vi "BusController.vi"() -> ()   [LabVIEW 2017, in "BusController.lvlib"]
uses:
  BusController.lvlib
  Admin/BCAdmin.lvclass
  Admin/BCAdmin.lvclass/BCAdmin.ctl
  Queue/QueueType.ctl
  Bus_class/Private/BdcstInfo.ctl
  Bus_class/Private/ModuleType.ctl
  Bus_class/Public/TypeDefs/clBusData.ctl
  FrontPanel/TypeDefs/clEventConfig.ctl
  Modules/PmuImpairPlugins/PmuImpairPluginBase_class/TypeDefs/clImpairConfig.ctl
  Modules/EventPlugins/EventPluginBaseClass/TypeDefs/clEvtReportArray.ctl
  Modules/EventPlugins/EventPluginBaseClass/TypeDefs/clEvtReport.ctl
  Modules/EventPlugins/EventPluginBaseClass/TypeDefs/dblEvtSignalArray.ctl
  Modules/NetworkImpairmentModule/PublicAPI/Arguments/Broadcasts/dblNetworkTime.ctl
  Modules/NetworkImpairmentModule/PublicAPI/Arguments/Broadcasts/dblPktLoss.ctl
  Modules/FlagImpairModule/PublicAPI/Arguments/Broadcasts/ui32FlagImpairmentArray.ctl
  Modules/OutputToFilePlugins/OutputToFileBasePlugin/Typedefs/PmuCfgOpt.ctl
  Admin/Accessors/Read ShowPanel_.vi
  Admin/Accessors/Read BC ID.vi
  Admin/Accessors/Read Name.vi
  Admin/Read Script.vi
  Admin/Accessors/Read BusIndex.vi
  Admin/Accessors/Read First_.vi
  Admin/Read BcQueName.vi
  Admin/Accessors/Read BCRegRef.vi
  <vilib>/Utility/error.llb/Error Cluster From Error Code.vi
  <vilib>/Analysis/1siggen.llb/Ramp Pattern by Delta.vi
  <vilib>/ErrorRing/Error Ring.xnode
  Admin/Registry/BCReg.lvclass
  Bus_class/Bus.lvclass
  <userlib>/NIST/NISTErrorLib/NISTErrorLib.lvlib
  Framework.lvlib
  Modules/PmuImpairPlugins/PmuImpairPluginBase_class/PmuImpairPluginBase.lvclass
  Modules/EventPlugins/EventPluginBaseClass/EventPluginBaseClass.lvclass
  Modules/NetworkImpairmentModule/NetworkImpairmentModule.lvlib
  Modules/FlagImpairModule/FlagImpairModule.lvlib
  Modules/OutputToFilePlugins/OutputToFileBasePlugin/OutputToFileBasePlugin.lvclass
  Modules/EventModule/EventModule.lvlib
  <vilib>/Analysis/NI_AALBase.lvlib
  Modules/PmuImpairModule/PmuImpairModule.lvlib
  ModuleType.ctl
panel:
  out "LastCommand":string
  out "Script":string[](array[string])
  out "BcQueName":string
  out "BC ID":i32
  out "First_":bool
  in  "BCAdmin":refnum<class "BCAdmin.lvclass">
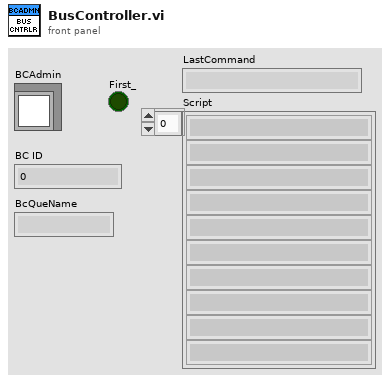
[diagram p1: front panel]
types:
  T1 = typedef "Framework.lvlib/clFrameworkData.ctl" = cluster{"EvtINIFilePaths":path[], "BusClassInstances":refnum<class "Bus.lvclass">[], "PmuImpairINIFilePaths":path[], "FlagImpairINIFilePaths":path[], "NetImpairINIFilePaths":path[], "OutputToFileINIFilePaths":path[], "AppINIFilePaths":path[], "AppModuleID":i32, "OutputToFileID":i32}
  T2 = typedef "Bus_class.lvlib/Bus.lvclass/ModuleType.ctl" = enum16{"PMU", "Event", "Network", "Flag", "App", "OutToFile"}
  T3 = typedef "Bus_class.lvlib/Bus.lvclass/BdcstInfo.ctl" = cluster{"ModuleType":T2, "ModuleID":i32, "UsrEvtRef":variant, "ScriptCmd":string}
  T4 = typedef "BusController.lvlib/ModuleType.ctl" = enum16{"PMU", "Event", "Network", "Flag", "App"}
  T5 = enum32{"Invalid", "Standard", "Closed", "Hidden", "Minimized", "Maximized"}
  T6 = typedef "Bus_class.lvlib/Bus.lvclass/clBusData.ctl" = cluster{"BusNumber":u8, "EvtPluginINIFilePath":path, "EvtParams":string[][], "EvtConfig":T7, "Start Time":dbl, "End Time":dbl, "PmuImpairPluginINIFilePath":path, "PmuImpairParams ":string[][], "PmuImpairConfig":T8, "NetImpPluginINIFilePath":path, "NetImpParams":string[][], "FlagImpPluginINIFilePath":path, "FlagImpParams":string[][], "EvtReportArray":T9, "EventSignalArray":T11, "ImpairReportArray":T9, "NetworkTime":T12, "PktLoss":T13, "FlagImpArray":T14, "OutputToFilePluginINIFilePath":path, "Output File Path":path, "clConfigOptions":T15, "AppPluginINIFilePath":path, "AppConfig":variant, "AppOutput":variant}
  T7 = typedef "Framework.lvlib/clEventConfig.ctl" = cluster{"UTC Time 0":timestamp, "Nominal Frequency":u16, "Reporting Rate":u16, "Fsamp":u32, "PosSeq":bool}
  T8 = typedef "PmuImpairPlugins.lvlib/PmuImpairPluginBase.lvclass/clImpairConfig.ctl" = cluster{"FilterType":string, "bPosSeq":bool}
  T9 = typedef "EventPlugins.lvlib/EventPluginBaseClass.lvclass/clEvtReportArray.ctl" = T10[]
  T10 = typedef "EventPlugins.lvlib/EventPluginBaseClass.lvclass/clEvtReport.ctl" = cluster{"Timestamp":dbl, "Synx":cdb[], "Freq":dbl, "ROCOF":dbl, "ID":i16}
  T11 = typedef "EventPlugins.lvlib/EventPluginBaseClass.lvclass/dblEvtSignalArray.ctl" = dbl[][]
  T12 = typedef "NetworkImpairmentModule.lvlib/dblNetworkTime.ctl" = dbl[]
  T13 = typedef "NetworkImpairmentModule.lvlib/dblPktLoss.ctl" = dbl[]
  T14 = typedef "FlagImpairModule.lvlib/ui32FlagImpairmentArray.ctl" = u32[]
  T15 = typedef "OutputToFilePlugins.lvlib/OutputToFileBasePlugin.lvclass/PmuCfgOpt.ctl" = cluster{"TIME_BASE":u64, "STN":string, "IDCODE":u16, "rdoPolRect":enum32{"Rectangular", "Polar"}, "rdoFloatInt":enum32{"Float", "Integer"}, "PHUNIT":u64, "rdoFreqDfreq":enum32{"Float", "Integer"}, "CHNAM":string[], "chkCfg2Prefix":bool}
  T16 = typedef "BusController.lvlib/QueueType.ctl" = cluster{"Msg":string, "Data":variant}
  T17 = typedef "EventModule.lvlib/clBroadcastEvents.ctl" = cluster{"DidInit":refnum<user-event>, "StatusUpdate":refnum<user-event>, "ErrorReport":refnum<user-event>, "DidStop":refnum<user-event>, "ReadEvtConfig":refnum<user-event>, "ReadTimeArray":refnum<user-event>, "ReadEvtParams":refnum<user-event>, "GetEvtReportArray":refnum<user-event>, "ReadPathToPlugin":refnum<user-event>, "GetEvtSignal":refnum<user-event>, "ReadBusNumber":refnum<user-event>}
  T18 = typedef "PmuImpairModule.lvlib/clBroadcastEvents.ctl" = cluster{"DidInit":refnum<user-event>, "StatusUpdate":refnum<user-event>, "ErrorReport":refnum<user-event>, "DidStop":refnum<user-event>, "ImpairConfig":refnum<user-event>, "ImpairParams":refnum<user-event>, "ImpairReports":refnum<user-event>, "PathToPlugin":refnum<user-event>, "BusNumber":refnum<user-event>}
  T19 = typedef "NetworkImpairmentModule.lvlib/clBroadcastEvents.ctl" = cluster{"DidInit":refnum<user-event>, "StatusUpdate":refnum<user-event>, "ErrorReport":refnum<user-event>, "DidStop":refnum<user-event>, "ReadNetImpParams":refnum<user-event>, "ReadLossThreshold":refnum<user-event>, "GetNetworkTime":refnum<user-event>, "GetPktLoss":refnum<user-event>, "ReadPathToPlugin":refnum<user-event>}
  T20 = typedef "FlagImpairModule.lvlib/clBroadcastEvents.ctl" = cluster{"DidInit":refnum<user-event>, "StatusUpdate":refnum<user-event>, "ErrorReport":refnum<user-event>, "DidStop":refnum<user-event>, "ReadFlagImpairConfig":refnum<user-event>, "ReadPluginINIFilePath":refnum<user-event>, "ReadFlagImpairParams":refnum<user-event>, "ReadTimeArray":refnum<user-event>, "GetFlagImpairment":refnum<user-event>}
  T21 = typedef "Rendezvous RefNum" = refnum<k1>
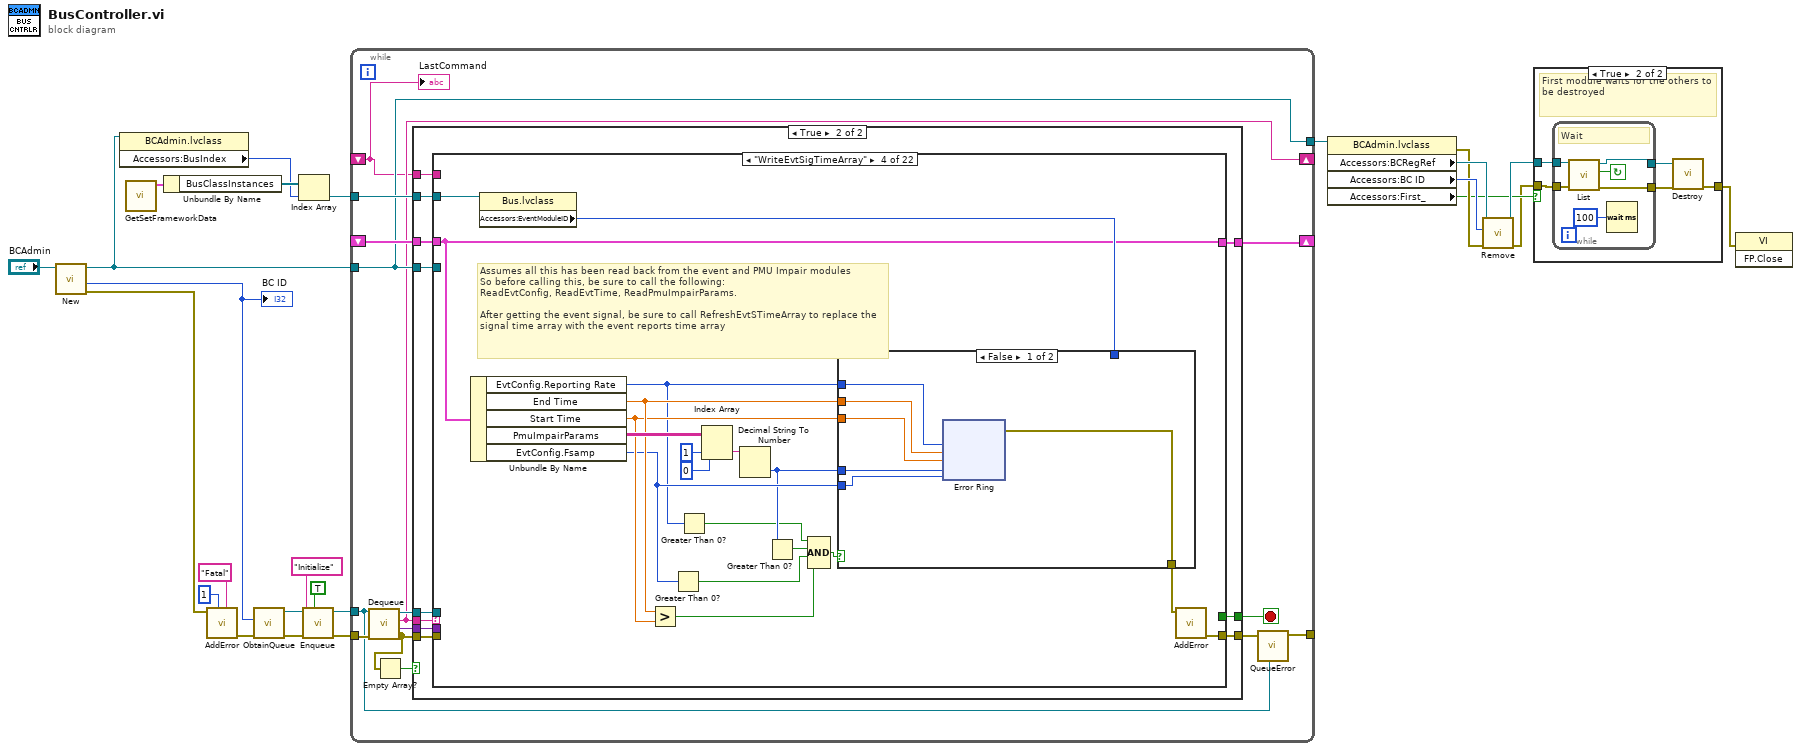
[diagram p0: block diagram]
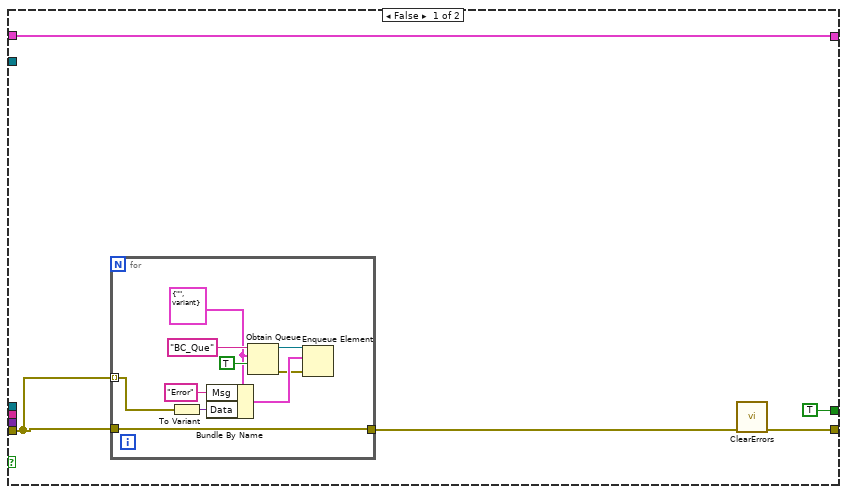
[diagram p3: hidden frame]
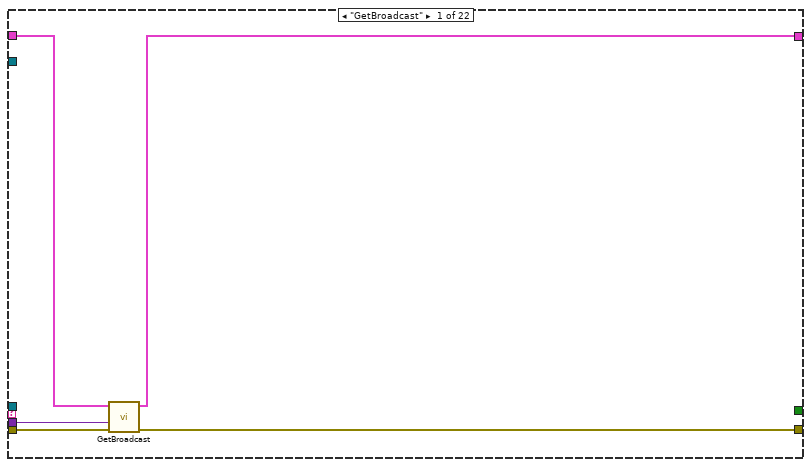
[diagram p4: hidden frame]
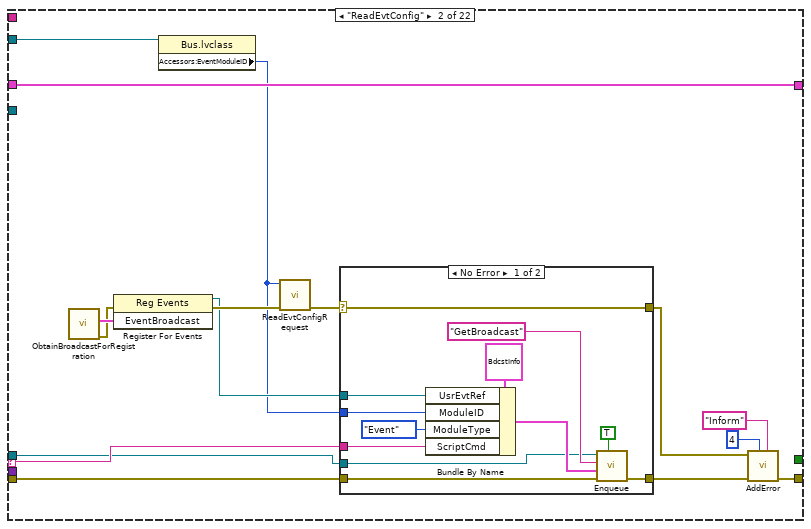
[diagram p5: hidden frame]
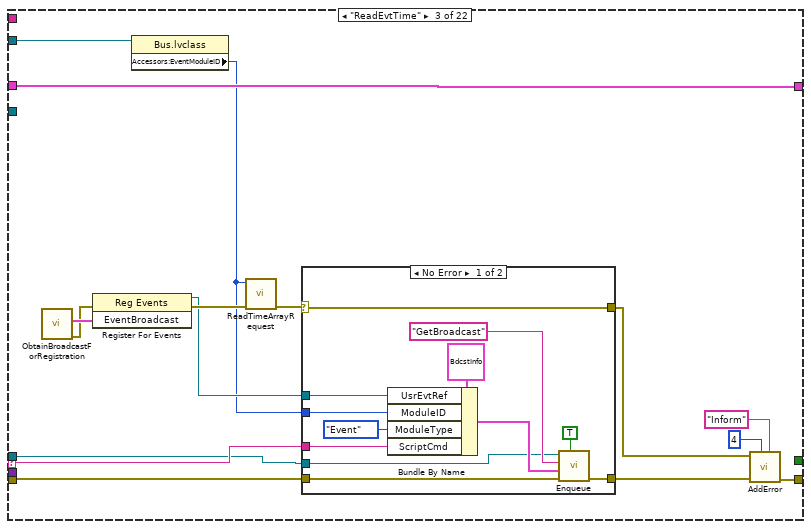
[diagram p7: hidden frame]
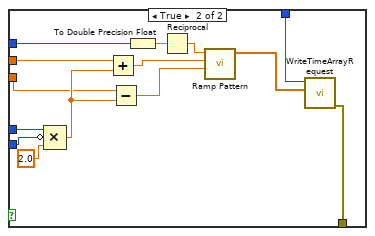
[diagram p9: hidden frame]
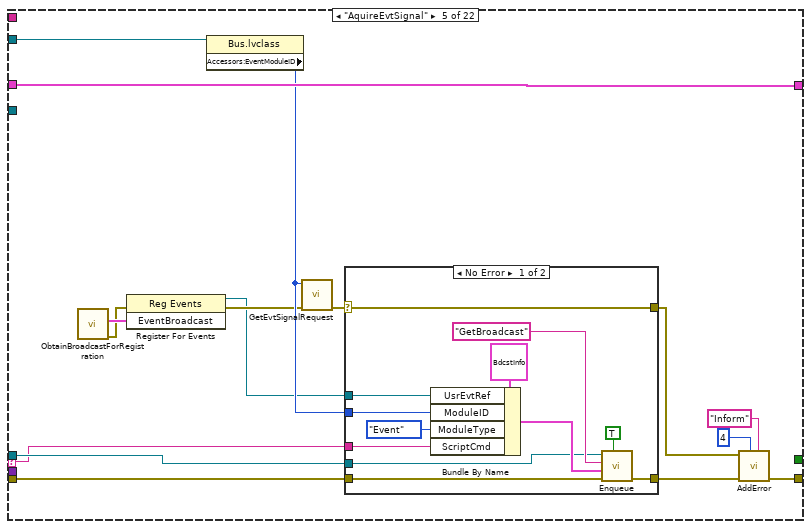
[diagram p10: hidden frame]
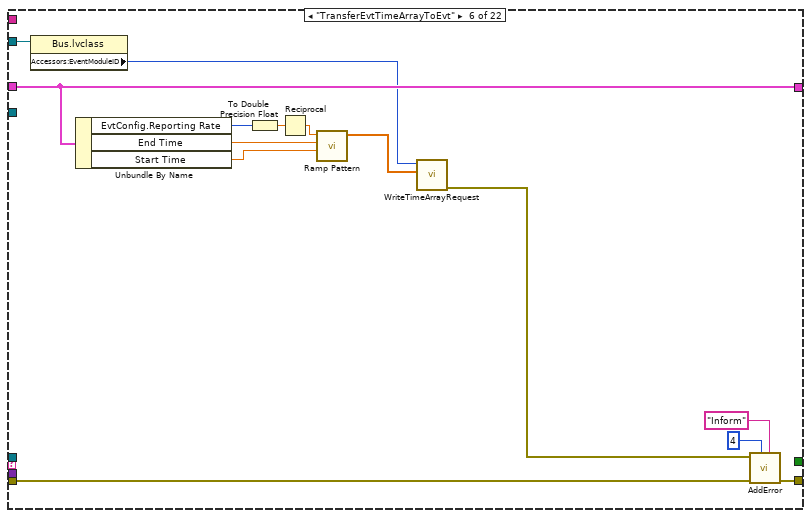
[diagram p12: hidden frame]
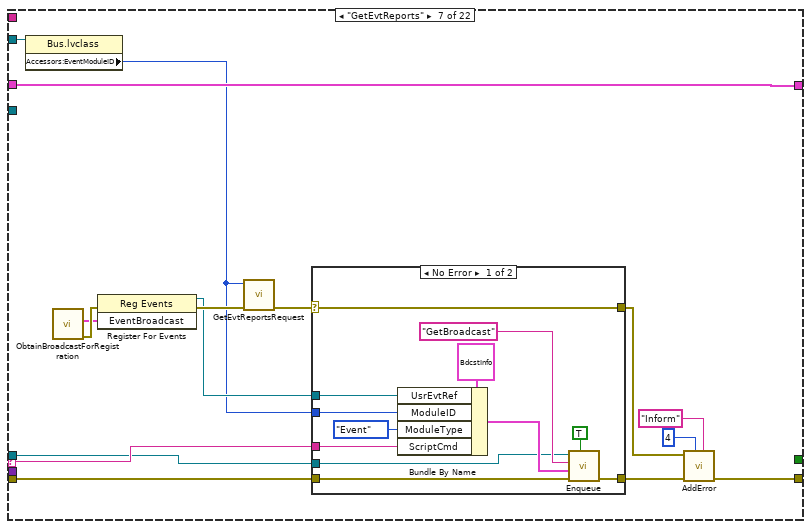
[diagram p13: hidden frame]
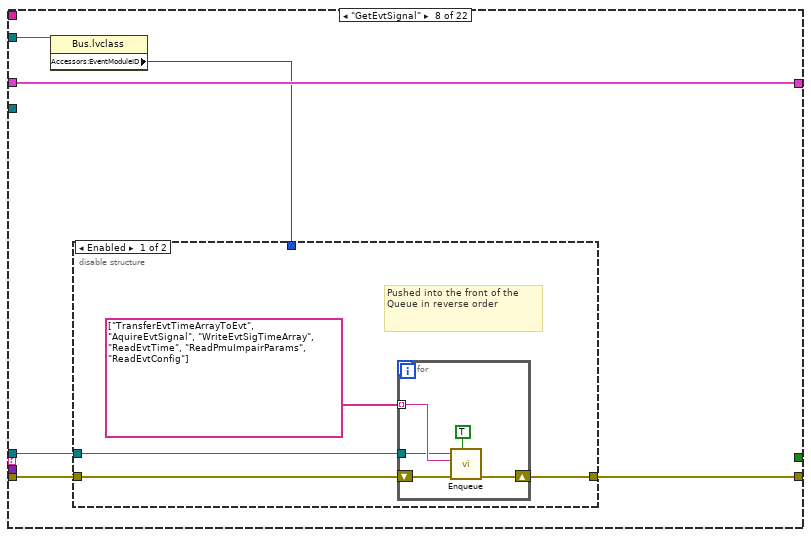
[diagram p15: hidden frame]
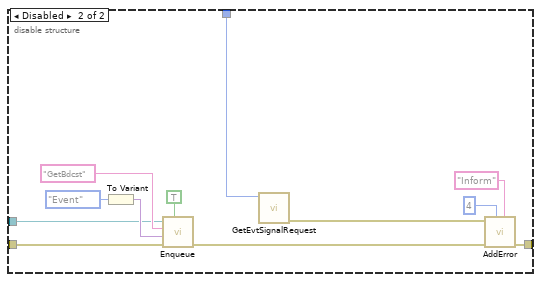
[diagram p16: hidden frame]
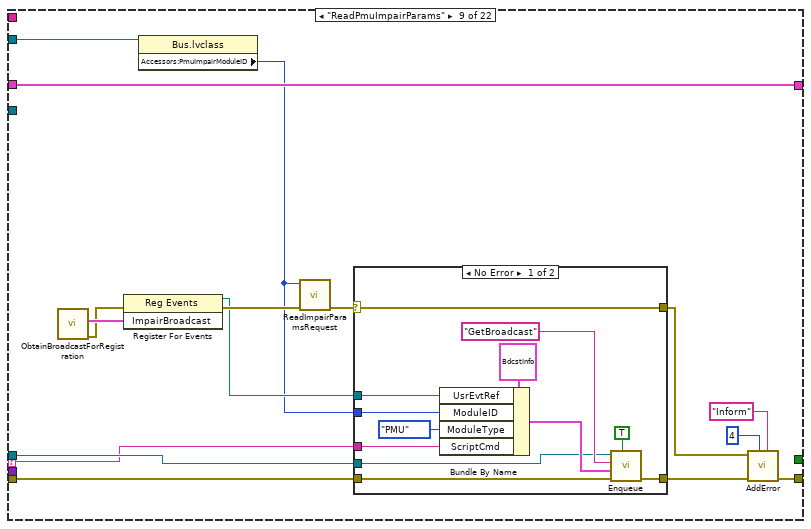
[diagram p17: hidden frame]
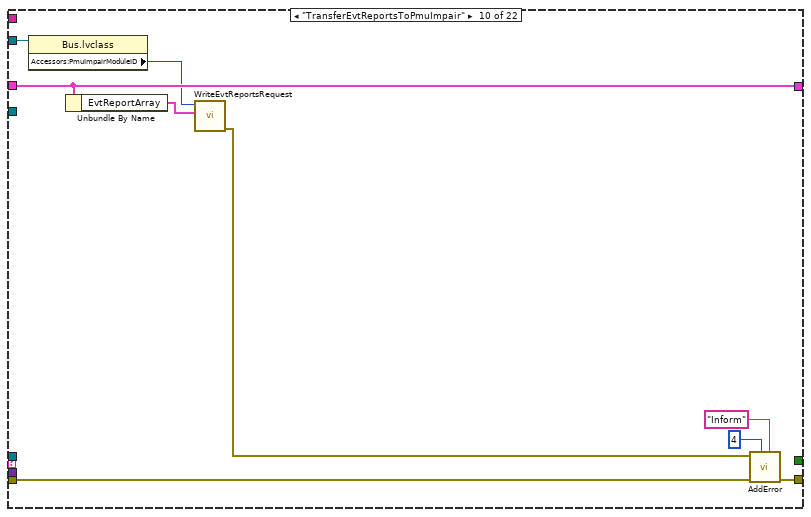
[diagram p19: hidden frame]
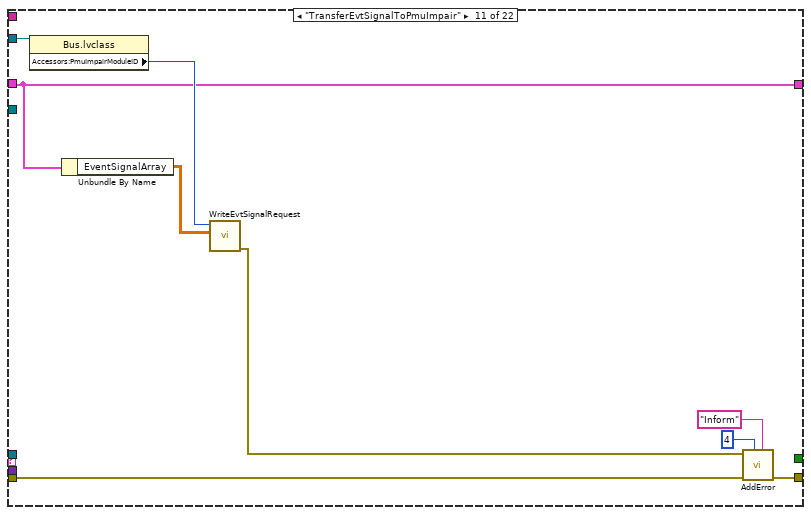
[diagram p20: hidden frame]
diagram:
  n1 = call "New.vi"("BCAdmin"="BCAdmin") -> ("error out"=w17:errorcluster, "BC ID"=w16:i32, "BCAdmin"=w7:refnum<class "BCAdmin.lvclass">)  [unwired: 7 in, 1 out]
  "BC ID" <- w16
  n2 = property class="BCAdmin.lvclass"(reference=w7) -> ("Accessors:BusIndex"=w4:u32)  [unwired: 1 in, 2 out]
  n3 = call "GetSetFrameworkData.vi"() -> ("clFrameworkData Out"=w5:T1)  [unwired: 11 in]
  n4 = Unbundle By Name(w5) -> ("BusClassInstances"=w6:refnum<class "Bus.lvclass">[])
  n5 = call <userlib>:"AddError.vi"("Severity"="Fatal", "Priority"=u8 1, "error in (no error)"=w17) -> ("ErrorArray"=w19:errorcluster[])  [unwired: 7 in, 1 out]
  n6 = call "ObtainQueue.vi"("Error In"=w19, "BC ID"=w16) -> ("Error Out"=w18:errorcluster[], "QueRef"=w2:refnum<queue>)  [unwired: 8 in]
  n7 = Index Array(array=w6, index=w4) -> (element=w3:refnum<class "Bus.lvclass">)
  n8 = call "Enqueue.vi"("Priority (f)"=TRUE, "Error In"=w18, "Msg"="Initialize", "QueRef"=w2) -> ("Error Out"=w24:errorcluster[], "QueRef"=w1:refnum<queue>)  [unwired: 6 in]
  n9 = while {
    tunnel: w7 -> [w33]
    tunnel: [w33] -> w15
    tunnel: w24 -> [w40]
    tunnel: [w37] -> _
    shift-right: [w26] -> _
    shift-left: _ -> [w35]
    tunnel: w3 -> [w34]
    tunnel: w1 -> [w29]
    shift-right: [w28] -> _
    shift-left: _ -> [w27]
    stop <- w36 stop-if-true
    n10 = call "Dequeue.vi"("Error In"=w40, "QueRef"=w29) -> ("Error Out"=w31:errorcluster[], "Data"=w39:variant, "Msg"=w28:string, "QueRef"=w30:refnum<queue>)  [unwired: 6 in]
    n11 = Empty Array?(array=w31) -> (empty?=w32:bool)
    n12 = case shown="True" w32 {
      tunnel: w31 -> [w42 w66]
      tunnel: w28 -> [_ w65]
      tunnel: w39 -> [_ w64]
      tunnel: [w44 w63] -> w38
      tunnel: [TRUE w62] -> w36
      tunnel: [w43 w61] -> w26
      tunnel: w35 -> [w43 w60]
      tunnel: w34 -> [_ w59]
      tunnel: w33 -> [_ w58]
      tunnel: w30 -> [_ w57]
      tunnel: w27 -> [_ w56]
      frame False {
        n13 = for {
          tunnel: w42 -> [w47] mode=indexing
          tunnel: [w46] -> w41
          tunnel: w42 -> [w46]
          w53 = T16 {"Msg"="", "Data"=variant} ("QueueType")
          n14 = To Variant(anything=w47) -> (Variant=w52:variant)
          n15 = Bundle By Name(cluster=w53, "Msg"="Error", "Data"=w52) -> (w50:T16)
          n16 = Obtain Queue(name (unnamed)="BC_Que", element data type=w53, create if not found? (T)=TRUE) -> (queue out=w51:refnum<queue>, error out=w49:errorcluster)  [unwired: 2 in, 1 out]
          n17 = Enqueue Element(queue=w51, element=w50, error in (no error)=w49) -> ()  [unwired: 1 in, 3 out]
        }
        n18 = call <userlib>:"ClearErrors.vi"("ErrorArray"=w41) -> ("ErrorArray"=w44:errorcluster[])  [unwired: 10 in]
      }
      frame True {
        n19 = case shown="\"WriteEvtSigTimeArray\"" w65 {
          selector: w65 -> [_ w73 w105 _ w189 _ w228 _ w289 _ _ w333 _ w382 w412 _ w456 _ _ _ _ w582]
          tunnel: w58 -> [_ _ _ _ _ _ _ _ _ _ _ _ _ _ _ _ _ w511 w559 _ _ w588]
          tunnel: w66 -> [w67 w74 w108 _ w192 w224 w235 w261 w293 w315 w324 w341 w365 w385 w415 w438 w459 w491 w545 w561 w563 w585]
          tunnel: [w68 w86 w116 w144 w196 w225 w238 w260 w297 w317 w326 w345 w366 w389 w419 w439 w463 w504 w549 w561 w568 w584] -> w63
          tunnel: w64 -> [w71 _ _ _ _ _ _ _ _ _ _ _ _ _ _ _ _ _ _ _ w567 _]
          tunnel: [_ _ _ _ _ _ _ _ _ _ _ _ _ _ _ _ _ _ _ TRUE _ _] -> w62
          tunnel: [w69 w83 w113 w142 w193 w215 w237 w259 w294 w320 w327 w342 w367 w386 w416 w441 w460 w488 w556 w560 w569 w583] -> w61
          tunnel: w60 -> [w70 w83 w113 w142 w193 w215 w237 w259 w294 w320 w327 w342 w367 w386 w416 w441 w460 _ w556 w560 w569 w583]
          tunnel: w59 -> [_ w87 w117 w146 w197 w213 w241 w257 w298 w321 w329 w346 w374 w390 w420 w448 w464 _ _ _ _ _]
          tunnel: w57 -> [_ w72 w104 _ w190 _ w227 w258 w290 _ _ w332 _ w381 w411 _ w455 w490 w542 _ _ _]
          tunnel: w56 -> [_ _ _ _ _ _ _ _ _ _ _ _ _ _ _ _ _ _ _ _ _ _]
          frame "GetBroadcast" {
            n20 = call "GetBroadcast.vi"("Error In"=w67, "BdcstInfo"=w71, "clBusData In"=w70) -> ("Error Out"=w68:errorcluster[], "clBusData Out"=w69:T6)  [unwired: 7 in]
          }
          frame "ReadEvtConfig" {
            n21 = call "ObtainBroadcastForRegistration.vi"() -> ("error out"=w81:errorcluster, "EventBroadcast"=w82:T17)  [unwired: 10 in]
            n22 = register-events(error in=w81, w82) -> (reference out=w76:refnum<event-registration>, error out=w80:errorcluster)  [unwired: 1 in]
            n23 = property class="Bus.lvclass"(reference=w87) -> ("Accessors:EventModuleID"=w75:i32)  [unwired: 1 in, 2 out]
            n24 = call "ReadEvtConfigRequest.vi"("error in (no error)"=w80, "ModuleID"=w75) -> ("error out"=w78:errorcluster)  [unwired: 9 in]
            n25 = case shown="No Error" w78 {
              selector: w78 -> [w93 w101]
              tunnel: [w96 w100] -> w79
              tunnel: [w93 w101] -> w77
              tunnel: w74 -> [w92 w100]
              tunnel: w75 -> [w91 _]
              tunnel: w76 -> [w90 _]
              tunnel: w73 -> [w89 _]
              tunnel: w72 -> [w88 _]
              frame No Error {
                n26 = Bundle By Name(cluster=T3 {"ModuleType"=enum."PMU", "ModuleID"=0, "UsrEvtRef"=variant, "ScriptCmd"=""} ("GetBdcstData"), "UsrEvtRef"=w90, "ModuleID"=w91, "ModuleType"=ModuleType."Event", "ScriptCmd"=w89) -> (w97:T3)
                n27 = call "Enqueue.vi"("Priority (f)"=TRUE, "Error In"=w92, "Data"=w97, "Msg"="GetBroadcast", "QueRef"=w88) -> ("Error Out"=w96:errorcluster[])  [unwired: 5 in, 1 out]
              }
              frame Error {
              }
            }
            n28 = call <userlib>:"AddError.vi"("Severity"="Inform", "Priority"=u8 4, "ErrorArray"=w79, "error in (no error)"=w77) -> ("ErrorArray"=w86:errorcluster[])  [unwired: 6 in, 1 out]
          }
          frame "ReadEvtTime" {
            n29 = call "ObtainBroadcastForRegistration.vi"() -> ("error out"=w110:errorcluster, "EventBroadcast"=w111:T17)  [unwired: 10 in]
            n30 = register-events(error in=w110, w111) -> (reference out=w107:refnum<event-registration>, error out=w109:errorcluster)  [unwired: 1 in]
            n31 = property class="Bus.lvclass"(reference=w117) -> ("Accessors:EventModuleID"=w106:i32)  [unwired: 1 in, 2 out]
            n32 = call "ReadTimeArrayRequest.vi"("error in (no error)"=w109, "ModuleID"=w106) -> ("error out"=w112:errorcluster)  [unwired: 9 in]
            n33 = case shown="No Error" w112 {
              selector: w112 -> [w123 w131]
              tunnel: [w126 w130] -> w103
              tunnel: [w123 w131] -> w102
              tunnel: w108 -> [w122 w130]
              tunnel: w106 -> [w121 _]
              tunnel: w107 -> [w120 _]
              tunnel: w105 -> [w119 _]
              tunnel: w104 -> [w118 _]
              frame No Error {
                n34 = Bundle By Name(cluster=T3 {"ModuleType"=enum."PMU", "ModuleID"=0, "UsrEvtRef"=variant, "ScriptCmd"=""} ("GetBdcstData"), "UsrEvtRef"=w120, "ModuleID"=w121, "ModuleType"=ModuleType."Event", "ScriptCmd"=w119) -> (w127:T3)
                n35 = call "Enqueue.vi"("Priority (f)"=TRUE, "Error In"=w122, "Data"=w127, "Msg"="GetBroadcast", "QueRef"=w118) -> ("Error Out"=w126:errorcluster[])  [unwired: 5 in, 1 out]
              }
              frame Error {
              }
            }
            n36 = call <userlib>:"AddError.vi"("Severity"="Inform", "Priority"=u8 4, "ErrorArray"=w103, "error in (no error)"=w102) -> ("ErrorArray"=w116:errorcluster[])  [unwired: 6 in, 1 out]
          }
          frame "WriteEvtSigTimeArray" {
            # "Assumes all this has been read back from the event and PMU Impair modules\nSo before calling this, be sure to call the following:\nReadEvtConfig, ReadEvtTime, ReadPmuImpairParams.\n\nAfter getting the event signal, be sure to call RefreshEvtSTimeArray to replace the signal time array with the event reports time array"
            n37 = Unbundle By Name(w142) -> ("EvtConfig.Reporting Rate"=w134:u16, "End Time"=w141:dbl, "Start Time"=w140:dbl, "PmuImpairParams"=w147:string[][], "EvtConfig.Fsamp"=w139:u32)
            n38 = property class="Bus.lvclass"(reference=w146) -> ("Accessors:EventModuleID"=w145:i32)  [unwired: 1 in, 2 out]
            n39 = Greater?(x=w141, y=w140) -> (0:w136:bool)
            n40 = Greater Than 0?(x=w139) -> (x > 0?=w137:bool)
            n41 = Greater Than 0?(x=w134) -> (x > 0?=w132:bool)
            n42 = Index Array(array=w147, index (row)=1, index (col)=0 ("disabled index (col)")) -> (element=w150:string)
            n43 = Decimal String To Number(string=w150) -> (number=w138:i32)  [unwired: 2 in, 1 out]
            n44 = Greater Than 0?(x=w138) -> (x > 0?=w133:bool)
            n45 = Compound Arithmetic op=AND(w132, w133, w137, w136) -> (w135:bool)
            n46 = case shown="False" w135 {
              tunnel: w134 -> [w156 w174]
              tunnel: w145 -> [_ w173]
              tunnel: [w151 w172] -> w143
              tunnel: w141 -> [w155 w171]
              tunnel: w140 -> [w154 w170]
              tunnel: w139 -> [w152 w169]
              tunnel: w138 -> [w153 w168]
              frame False {
                n47 = xnode "Error Ring"("parameter 0"=w156, "parameter 1"=w155, "parameter 2"=w154, "parameter 3"=w153, "parameter 4"=w152) -> ("error out"=w151:errorcluster)
              }
              frame True {
                n48 = Compound Arithmetic op=MULTIPLY(w168, invert w169, 2.0 ("value")) -> (w180:dbl)
                n49 = Add(x=w171, y=w180) -> (x+y=w179:dbl)
                n50 = Subtract(x=w170, y=w180) -> (x-y=w178:dbl)
                n51 = To Double Precision Float(number=w174) -> (double precision float=w175:dbl)
                n52 = Reciprocal(x=w175) -> (1/x=w176:dbl)
                n53 = call-poly <vilib>:"Ramp Pattern.vi"("start"=w178, "end"=w179, "delta"=w176) -> ("Ramp Pattern"=w177:dbl[])  [unwired: 6 in, 2 out]
                n54 = call "WriteTimeArrayRequest.vi"("TimeArray"=w177, "ModuleID"=w173) -> ("error out"=w172:errorcluster)  [unwired: 9 in]
              }
            }
            n55 = call <userlib>:"AddError.vi"("error in (no error)"=w143) -> ("ErrorArray"=w144:errorcluster[])  [unwired: 9 in, 1 out]
          }
          frame "AquireEvtSignal" {
            n56 = call "ObtainBroadcastForRegistration.vi"() -> ("error out"=w186:errorcluster, "EventBroadcast"=w187:T17)  [unwired: 10 in]
            n57 = register-events(error in=w186, w187) -> (reference out=w184:refnum<event-registration>, error out=w185:errorcluster)  [unwired: 1 in]
            n58 = property class="Bus.lvclass"(reference=w197) -> ("Accessors:EventModuleID"=w188:i32)  [unwired: 1 in, 2 out]
            n59 = call "GetEvtSignalRequest.vi"("error in (no error)"=w185, "ModuleID"=w188) -> ("error out"=w183:errorcluster)  [unwired: 9 in]
            n60 = case shown="No Error" w183 {
              selector: w183 -> [w203 w211]
              tunnel: [w206 w210] -> w191
              tunnel: [w203 w211] -> w182
              tunnel: w192 -> [w202 w210]
              tunnel: w188 -> [w201 _]
              tunnel: w184 -> [w200 _]
              tunnel: w189 -> [w199 _]
              tunnel: w190 -> [w198 _]
              frame No Error {
                n61 = Bundle By Name(cluster=T3 {"ModuleType"=enum."PMU", "ModuleID"=0, "UsrEvtRef"=variant, "ScriptCmd"=""} ("GetBdcstData"), "UsrEvtRef"=w200, "ModuleID"=w201, "ModuleType"=ModuleType."Event", "ScriptCmd"=w199) -> (w207:T3)
                n62 = call "Enqueue.vi"("Priority (f)"=TRUE, "Error In"=w202, "Data"=w207, "Msg"="GetBroadcast", "QueRef"=w198) -> ("Error Out"=w206:errorcluster[])  [unwired: 5 in, 1 out]
              }
              frame Error {
              }
            }
            n63 = call <userlib>:"AddError.vi"("Severity"="Inform", "Priority"=u8 4, "ErrorArray"=w191, "error in (no error)"=w182) -> ("ErrorArray"=w196:errorcluster[])  [unwired: 6 in, 1 out]
          }
          frame "TransferEvtTimeArrayToEvt" {
            n64 = property class="Bus.lvclass"(reference=w213) -> ("Accessors:EventModuleID"=w212:i32)  [unwired: 1 in, 2 out]
            n65 = Unbundle By Name(w215) -> ("EvtConfig.Reporting Rate"=w221:u16, "End Time"=w217:dbl, "Start Time"=w216:dbl)
            n66 = To Double Precision Float(number=w221) -> (double precision float=w220:dbl)
            n67 = Reciprocal(x=w220) -> (1/x=w219:dbl)
            n68 = call-poly <vilib>:"Ramp Pattern.vi"("start"=w216, "end"=w217, "delta"=w219) -> ("Ramp Pattern"=w218:dbl[])  [unwired: 6 in, 2 out]
            n69 = call "WriteTimeArrayRequest.vi"("TimeArray"=w218, "ModuleID"=w212) -> ("error out"=w214:errorcluster)  [unwired: 9 in]
            n70 = call <userlib>:"AddError.vi"("Severity"="Inform", "Priority"=u8 4, "ErrorArray"=w224, "error in (no error)"=w214) -> ("ErrorArray"=w225:errorcluster[])  [unwired: 6 in, 1 out]
          }
          frame "GetEvtReports" {
            n71 = property class="Bus.lvclass"(reference=w241) -> ("Accessors:EventModuleID"=w229:i32)  [unwired: 1 in, 2 out]
            n72 = call "ObtainBroadcastForRegistration.vi"() -> ("error out"=w233:errorcluster, "EventBroadcast"=w232:T17)  [unwired: 10 in]
            n73 = register-events(error in=w233, w232) -> (reference out=w230:refnum<event-registration>, error out=w231:errorcluster)  [unwired: 1 in]
            n74 = call "GetEvtReportsRequest.vi"("error in (no error)"=w231, "ModuleID"=w229) -> ("error out"=w234:errorcluster)  [unwired: 9 in]
            n75 = case shown="No Error" w234 {
              selector: w234 -> [w247 w255]
              tunnel: [w250 w254] -> w236
              tunnel: [w247 w255] -> w226
              tunnel: w235 -> [w246 w254]
              tunnel: w229 -> [w245 _]
              tunnel: w230 -> [w244 _]
              tunnel: w228 -> [w243 _]
              tunnel: w227 -> [w242 _]
              frame No Error {
                n76 = Bundle By Name(cluster=T3 {"ModuleType"=enum."PMU", "ModuleID"=0, "UsrEvtRef"=variant, "ScriptCmd"=""} ("GetBdcstData"), "UsrEvtRef"=w244, "ModuleID"=w245, "ModuleType"=ModuleType."Event", "ScriptCmd"=w243) -> (w251:T3)
                n77 = call "Enqueue.vi"("Priority (f)"=TRUE, "Error In"=w246, "Data"=w251, "Msg"="GetBroadcast", "QueRef"=w242) -> ("Error Out"=w250:errorcluster[])  [unwired: 5 in, 1 out]
              }
              frame Error {
              }
            }
            n78 = call <userlib>:"AddError.vi"("Severity"="Inform", "Priority"=u8 4, "ErrorArray"=w236, "error in (no error)"=w226) -> ("ErrorArray"=w238:errorcluster[])  [unwired: 6 in, 1 out]
          }
          frame "GetEvtSignal" {
            n79 = property class="Bus.lvclass"(reference=w257) -> ("Accessors:EventModuleID"=w256:i32)  [unwired: 1 in, 2 out]
            n80 = disable-structure shown="Enabled" {
              disable-tunnel: w261 -> [w264 w273]
              disable-tunnel: [w263 w281] -> w260
              disable-tunnel: w258 -> [w262 w271]
              disable-tunnel: w256 -> [_ w282]
              frame Enabled {
                # "Pushed into the front of the Queue in reverse order"
                n81 = for {
                  tunnel: string[] ["TransferEvtTimeArrayToEvt", "AquireEvtSignal", "WriteEvtSigTimeArray", "ReadEvtTime", "ReadPmuImpairParams", "ReadEvtConfig"] -> [w270] mode=indexing
                  shift-right: [w268] -> w263
                  shift-left: w264 -> [w269]
                  tunnel: w262 -> [w266]
                  n82 = call "Enqueue.vi"("Priority (f)"=TRUE, "Error In"=w269, "Msg"=w270, "QueRef"=w266) -> ("Error Out"=w268:errorcluster[])  [unwired: 6 in, 1 out]
                }
              }
              frame Disabled {
                n83 = To Variant(anything=ModuleType."Event" ("ModuleType")) -> (Variant=w276:variant)
                n84 = call "Enqueue.vi"("Priority (f)"=TRUE, "Error In"=w273, "Data"=w276, "Msg"="GetBdcst", "QueRef"=w271) -> ("Error Out"=w272:errorcluster[])  [unwired: 5 in, 1 out]
                n85 = call "GetEvtSignalRequest.vi"("ModuleID"=w282) -> ("error out"=w280:errorcluster)  [unwired: 10 in]
                n86 = call <userlib>:"AddError.vi"("Severity"="Inform", "Priority"=u8 4, "ErrorArray"=w272, "error in (no error)"=w280) -> ("ErrorArray"=w281:errorcluster[])  [unwired: 6 in, 1 out]
              }
            }
          }
          frame "ReadPmuImpairParams" {
            n87 = call "ObtainBroadcastForRegistration.vi"() -> ("error out"=w286:errorcluster, "ImpairBroadcast"=w287:T18)  [unwired: 10 in]
            n88 = register-events(error in=w286, w287) -> (reference out=w284:refnum<event-registration>, error out=w285:errorcluster)  [unwired: 1 in]
            n89 = property class="Bus.lvclass"(reference=w298) -> ("Accessors:PmuImpairModuleID"=w283:i32)  [unwired: 1 in, 2 out]
            n90 = call "ReadImpairParamsRequest.vi"("error in (no error)"=w285, "ModuleID"=w283) -> ("error out"=w288:errorcluster)  [unwired: 9 in]
            n91 = case shown="No Error" w288 {
              selector: w288 -> [w304 w312]
              tunnel: [w307 w311] -> w292
              tunnel: [w304 w312] -> w291
              tunnel: w293 -> [w303 w311]
              tunnel: w283 -> [w302 _]
              tunnel: w284 -> [w301 _]
              tunnel: w289 -> [w300 _]
              tunnel: w290 -> [w299 _]
              frame No Error {
                n92 = Bundle By Name(cluster=T3 {"ModuleType"=enum."PMU", "ModuleID"=0, "UsrEvtRef"=variant, "ScriptCmd"=""} ("GetBdcstData"), "UsrEvtRef"=w301, "ModuleID"=w302, "ModuleType"=ModuleType."PMU", "ScriptCmd"=w300) -> (w308:T3)
                n93 = call "Enqueue.vi"("Priority (f)"=TRUE, "Error In"=w303, "Data"=w308, "Msg"="GetBroadcast", "QueRef"=w299) -> ("Error Out"=w307:errorcluster[])  [unwired: 5 in, 1 out]
              }
              frame Error {
              }
            }
            n94 = call <userlib>:"AddError.vi"("Severity"="Inform", "Priority"=u8 4, "ErrorArray"=w292, "error in (no error)"=w291) -> ("ErrorArray"=w297:errorcluster[])  [unwired: 6 in, 1 out]
          }
          frame "TransferEvtReportsToPmuImpair" {
            n95 = property class="Bus.lvclass"(reference=w321) -> ("Accessors:PmuImpairModuleID"=w319:i32)  [unwired: 1 in, 2 out]
            n96 = Unbundle By Name(w320) -> ("EvtReportArray"=w318:T9)
            n97 = call "WriteEvtReportsRequest.vi"("EvtReportArray"=w318, "ModuleID"=w319) -> ("error out"=w316:errorcluster)  [unwired: 9 in]
            n98 = call <userlib>:"AddError.vi"("Severity"="Inform", "Priority"=u8 4, "ErrorArray"=w315, "error in (no error)"=w316) -> ("ErrorArray"=w317:errorcluster[])  [unwired: 6 in, 1 out]
          }
          frame "TransferEvtSignalToPmuImpair" {
            n99 = property class="Bus.lvclass"(reference=w329) -> ("Accessors:PmuImpairModuleID"=w328:i32)  [unwired: 1 in, 2 out]
            n100 = Unbundle By Name(w327) -> ("EventSignalArray"=w330:T11)
            n101 = call "WriteEvtSignalRequest.vi"("EvtSignalArray"=w330, "ModuleID"=w328) -> ("error out"=w325:errorcluster)  [unwired: 9 in]
            n102 = call <userlib>:"AddError.vi"("Severity"="Inform", "Priority"=u8 4, "ErrorArray"=w324, "error in (no error)"=w325) -> ("ErrorArray"=w326:errorcluster[])  [unwired: 6 in, 1 out]
          }
          frame "GetPmuImpairReports" {
            n103 = call "ObtainBroadcastForRegistration.vi"() -> ("error out"=w338:errorcluster, "ImpairBroadcast"=w337:T18)  [unwired: 10 in]
            n104 = register-events(error in=w338, w337) -> (reference out=w335:refnum<event-registration>, error out=w336:errorcluster)  [unwired: 1 in]
            n105 = property class="Bus.lvclass"(reference=w346) -> ("Accessors:PmuImpairModuleID"=w334:i32)  [unwired: 1 in, 2 out]
            n106 = call "GetImpairReportsRequest.vi"("error in (no error)"=w336, "ModuleID"=w334) -> ("error out"=w339:errorcluster)  [unwired: 9 in]
            n107 = case shown="No Error" w339 {
              selector: w339 -> [w352 w360]
              tunnel: [w355 w359] -> w340
              tunnel: [w352 w360] -> w331
              tunnel: w341 -> [w351 w359]
              tunnel: w334 -> [w350 _]
              tunnel: w335 -> [w349 _]
              tunnel: w333 -> [w348 _]
              tunnel: w332 -> [w347 _]
              frame No Error {
                n108 = Bundle By Name(cluster=T3 {"ModuleType"=enum."PMU", "ModuleID"=0, "UsrEvtRef"=variant, "ScriptCmd"=""} ("GetBdcstData"), "UsrEvtRef"=w349, "ModuleID"=w350, "ModuleType"=ModuleType."PMU", "ScriptCmd"=w348) -> (w356:T3)
                n109 = call "Enqueue.vi"("Priority (f)"=TRUE, "Error In"=w351, "Data"=w356, "Msg"="GetBroadcast", "QueRef"=w347) -> ("Error Out"=w355:errorcluster[])  [unwired: 5 in, 1 out]
              }
              frame Error {
              }
            }
            n110 = call <userlib>:"AddError.vi"("Severity"="Inform", "Priority"=u8 4, "ErrorArray"=w340, "error in (no error)"=w331) -> ("ErrorArray"=w345:errorcluster[])  [unwired: 6 in, 1 out]
          }
          frame "TransferTimeArrayToNetImpair" {
            n111 = property class="Bus.lvclass"(reference=w374) -> ("Accessors:NetworkImpairModuleID"=w363:i32)  [unwired: 1 in, 2 out]
            n112 = Unbundle By Name(w367) -> ("EvtConfig.Reporting Rate"=w370:u16, "End Time"=w371:dbl, "Start Time"=w372:dbl)
            n113 = To Double Precision Float(number=w370) -> (double precision float=w368:dbl)
            n114 = Reciprocal(x=w368) -> (1/x=w369:dbl)
            n115 = call-poly <vilib>:"Ramp Pattern.vi"("start"=w372, "end"=w371, "delta"=w369) -> ("Ramp Pattern"=w373:dbl[])  [unwired: 6 in, 2 out]
            n116 = call "WriteTimeArrayRequest.vi"("TimeArray"=w373, "Module ID"=w363) -> ("error out"=w364:errorcluster)  [unwired: 9 in]
            n117 = call <userlib>:"AddError.vi"("Severity"="Inform", "Priority"=u8 4, "ErrorArray"=w365, "error in (no error)"=w364) -> ("ErrorArray"=w366:errorcluster[])  [unwired: 6 in, 1 out]
          }
          frame "GetNetImpairTime" {
            n118 = call "ObtainBroadcastForRegistration.vi"() -> ("error out"=w378:errorcluster, "NetImpBroadcast"=w379:T19)  [unwired: 10 in]
            n119 = register-events(error in=w378, w379) -> (reference out=w383:refnum<event-registration>, error out=w376:errorcluster)  [unwired: 1 in]
            n120 = property class="Bus.lvclass"(reference=w390) -> ("Accessors:PmuImpairModuleID"=w375:i32)  [unwired: 1 in, 2 out]
            n121 = call "GetNetTimeRequest.vi"("error in (no error)"=w376, "ModuleID"=w375) -> ("error out"=w377:errorcluster)  [unwired: 9 in]
            n122 = case shown="No Error" w377 {
              selector: w377 -> [w396 w404]
              tunnel: [w399 w403] -> w384
              tunnel: [w396 w404] -> w380
              tunnel: w385 -> [w395 w403]
              tunnel: w375 -> [w394 _]
              tunnel: w383 -> [w393 _]
              tunnel: w382 -> [w392 _]
              tunnel: w381 -> [w391 _]
              frame No Error {
                n123 = Bundle By Name(cluster=T3 {"ModuleType"=enum."PMU", "ModuleID"=0, "UsrEvtRef"=variant, "ScriptCmd"=""} ("GetBdcstData"), "UsrEvtRef"=w393, "ModuleID"=w394, "ModuleType"=ModuleType."Network", "ScriptCmd"=w392) -> (w400:T3)
                n124 = call "Enqueue.vi"("Priority (f)"=TRUE, "Error In"=w395, "Data"=w400, "Msg"="GetBroadcast", "QueRef"=w391) -> ("Error Out"=w399:errorcluster[])  [unwired: 5 in, 1 out]
              }
              frame Error {
              }
            }
            n125 = call <userlib>:"AddError.vi"("Severity"="Inform", "Priority"=u8 4, "ErrorArray"=w384, "error in (no error)"=w380) -> ("ErrorArray"=w389:errorcluster[])  [unwired: 6 in, 1 out]
          }
          frame "GetNetPktLoss" {
            n126 = call "ObtainBroadcastForRegistration.vi"() -> ("error out"=w408:errorcluster, "NetImpBroadcast"=w409:T19)  [unwired: 10 in]
            n127 = register-events(error in=w408, w409) -> (reference out=w413:refnum<event-registration>, error out=w406:errorcluster)  [unwired: 1 in]
            n128 = property class="Bus.lvclass"(reference=w420) -> ("Accessors:NetworkImpairModuleID"=w405:i32)  [unwired: 1 in, 2 out]
            n129 = call "GetPktLossRequest.vi"("error in (no error)"=w406, "ModuleID"=w405) -> ("error out"=w407:errorcluster)  [unwired: 9 in]
            n130 = case shown="No Error" w407 {
              selector: w407 -> [w426 w434]
              tunnel: [w429 w433] -> w414
              tunnel: [w426 w434] -> w410
              tunnel: w415 -> [w425 w433]
              tunnel: w405 -> [w424 _]
              tunnel: w413 -> [w423 _]
              tunnel: w412 -> [w422 _]
              tunnel: w411 -> [w421 _]
              frame No Error {
                n131 = Bundle By Name(cluster=T3 {"ModuleType"=enum."PMU", "ModuleID"=0, "UsrEvtRef"=variant, "ScriptCmd"=""} ("GetBdcstData"), "UsrEvtRef"=w423, "ModuleID"=w424, "ModuleType"=ModuleType."Network", "ScriptCmd"=w422) -> (w430:T3)
                n132 = call "Enqueue.vi"("Priority (f)"=TRUE, "Error In"=w425, "Data"=w430, "Msg"="GetBroadcast", "QueRef"=w421) -> ("Error Out"=w429:errorcluster[])  [unwired: 5 in, 1 out]
              }
              frame Error {
              }
            }
            n133 = call <userlib>:"AddError.vi"("Severity"="Inform", "Priority"=u8 4, "ErrorArray"=w414, "error in (no error)"=w410) -> ("ErrorArray"=w419:errorcluster[])  [unwired: 6 in, 1 out]
          }
          frame "TransferTimeArrayToFlagImpair" {
            n134 = property class="Bus.lvclass"(reference=w448) -> ("Accessors:FlagImpairModuleID"=w440:i32)  [unwired: 1 in, 2 out]
            n135 = Unbundle By Name(w441) -> ("EvtConfig.Reporting Rate"=w444:u16, "End Time"=w445:dbl, "Start Time"=w446:dbl)
            n136 = To Double Precision Float(number=w444) -> (double precision float=w442:dbl)
            n137 = Reciprocal(x=w442) -> (1/x=w443:dbl)
            n138 = call-poly <vilib>:"Ramp Pattern.vi"("start"=w446, "end"=w445, "delta"=w443) -> ("Ramp Pattern"=w447:dbl[])  [unwired: 6 in, 2 out]
            n139 = call "WriteTimeArrayRequest.vi"("dblTimeArray"=w447, "ModuleID"=w440) -> ("error out"=w437:errorcluster)  [unwired: 9 in]
            n140 = call <userlib>:"AddError.vi"("Severity"="Inform", "Priority"=u8 4, "ErrorArray"=w438, "error in (no error)"=w437) -> ("ErrorArray"=w439:errorcluster[])  [unwired: 6 in, 1 out]
          }
          frame "GetFlagImpairArray" {
            n141 = call "ObtainBroadcastForRegistration.vi"() -> ("error out"=w452:errorcluster, "FlagImpairBroadcasts"=w453:T20)  [unwired: 10 in]
            n142 = register-events(error in=w452, w453) -> (reference out=w457:refnum<event-registration>, error out=w450:errorcluster)  [unwired: 1 in]
            n143 = property class="Bus.lvclass"(reference=w464) -> ("Accessors:FlagImpairModuleID"=w449:i32)  [unwired: 1 in, 2 out]
            n144 = call "GetFlagImpairmentArrayRequest.vi"("error in (no error)"=w450, "ModuleID"=w449) -> ("error out"=w451:errorcluster)  [unwired: 9 in]
            n145 = case shown="No Error" w451 {
              selector: w451 -> [w470 w478]
              tunnel: [w473 w477] -> w458
              tunnel: [w470 w478] -> w454
              tunnel: w459 -> [w469 w477]
              tunnel: w449 -> [w468 _]
              tunnel: w457 -> [w467 _]
              tunnel: w456 -> [w466 _]
              tunnel: w455 -> [w465 _]
              frame No Error {
                n146 = Bundle By Name(cluster=T3 {"ModuleType"=enum."PMU", "ModuleID"=0, "UsrEvtRef"=variant, "ScriptCmd"=""} ("GetBdcstData"), "UsrEvtRef"=w467, "ModuleID"=w468, "ModuleType"=ModuleType."Flag", "ScriptCmd"=w466) -> (w474:T3)
                n147 = call "Enqueue.vi"("Priority (f)"=TRUE, "Error In"=w469, "Data"=w474, "Msg"="GetBroadcast", "QueRef"=w465) -> ("Error Out"=w473:errorcluster[])  [unwired: 5 in, 1 out]
              }
              frame Error {
              }
            }
            n148 = call <userlib>:"AddError.vi"("Severity"="Inform", "Priority"=u8 4, "ErrorArray"=w458, "error in (no error)"=w454) -> ("ErrorArray"=w463:errorcluster[])  [unwired: 6 in, 1 out]
          }
          frame "Initialize" {
            # "Error Check:\nQue should \nbe empty"
            n149 = property class="BCAdmin.lvclass"(reference=w511) -> (error out=w509:errorcluster, "Accessors:ShowPanel_"=w481:bool, "Accessors:BC ID"=w483:i32, "Accessors:Name"=w484:string, "Accessors:Script"=w485:string[], "Accessors:BusIndex"=w486:u32, "Accessors:First_"=→"First_":bool)  [unwired: 1 in, 1 out]
            "Script" <- w485
            n150 = Get Queue Status(queue=w490) -> (queue out=w489:refnum<queue>, # elements in queue=w510:i32)  [unwired: 2 in, 6 out]
            n151 = case shown="0" w510 {
              tunnel: w483 -> [_ w534]
              tunnel: w491 -> [w515 w530]
              tunnel: [w513 w529] -> w503
              tunnel: w485 -> [w514 _]
              tunnel: w489 -> [w512 _]
              frame 0 {
                n152 = for {
                  shift-right: [w520] -> w513
                  shift-left: w515 -> [w521]
                  tunnel: w514 -> [w522] mode=indexing
                  tunnel: w512 -> [w516]
                  n153 = Spreadsheet String To Array(delimiter (Tab)="," ("format string"), format string="%s", spreadsheet string=w522, array type (2D Dbl)=string[] []) -> (array=w525:string[])
                  n154 = Split 1D Array(array=w525, index=1) -> (first subarray=w528:string[], second subarray=w527:string[])
                  n155 = To Variant(anything=w527) -> (Variant=w519:variant)
                  n156 = Index Array(array=w528) -> (element=w517:string)  [unwired: 1 in]
                  n157 = call "Enqueue.vi"("Error In"=w521, "Data"=w519, "Msg"=w517, "QueRef"=w516) -> ("Error Out"=w520:errorcluster[])  [unwired: 6 in, 1 out]
                }
              }
              frame 1, Default {
                n158 = xnode "Error Ring"("parameter 0"=w534) -> ("error out"=w533:errorcluster)
                n159 = call <userlib>:"AddError.vi"("Severity"="Abort", "Priority"=u8 3, "ErrorArray"=w530, "error in (no error)"=w533) -> ("ErrorArray"=w529:errorcluster[])  [unwired: 6 in, 1 out]
              }
            }
            n160 = Select(t=T5."Standard" ("State"), s=w481, f=T5."Hidden" ("State")) -> (s? t:f=w479:T5)
            n161 = invoke class="VI" method="FP.Open"(error in=w509, "State"=w479) -> (reference out=w508:refnum<vi>, error out=w507:errorcluster)  [unwired: 3 in, 3 out]
            n162 = property class="VI"(reference=w508, error in=w507, "Front Panel.Title"=w484) -> (reference out=w505:refnum<vi>, error out=w506:errorcluster)
            n163 = Increment(x=w486) -> (x+1=w499:u32)
            n164 = invoke class="VI" method="FP.Center"(reference=w505, error in=w506) -> (error out=w496:errorcluster)  [unwired: 1 in, 2 out]
            n165 = call <vilib>:"Create Rendezvous.vi"("error in (no error)"=w496, "return existing (F)"=TRUE, "name (unnamed)"="BC_Rndz") -> ("error out"=w495:errorcluster, "rendezvous"=w492:T21)  [unwired: 2 in, 1 out]
            n166 = Bundle By Name(cluster=T6 {"BusNumber"=0, "EvtPluginINIFilePath"=path "", "EvtParams"=[], "EvtConfig"={"UTC Time 0"=timestamp(0 s since 1904-01-01), "Nominal Frequency"=60, "Reporting Rate"=60, "Fsamp"=960, "PosSeq"=FALSE}, "Start Time"=0.0, "End Time"=0.0, "PmuImpairPluginINIFilePath"=path "", "PmuImpairParams "=[["960"], ["8.19"], ["164"]], "PmuImpairConfig"={"FilterType"="", "bPosSeq"=TRUE}, "NetImpPluginINIFilePath"=path "", "NetImpParams"=[], "FlagImpPluginINIFilePath"=path "", "FlagImpParams"=[], "EvtReportArray"=[], "EventSignalArray"=[], "ImpairReportArray"=[], "NetworkTime"=[], "PktLoss"=[], "FlagImpArray"=[], "OutputToFilePluginINIFilePath"=path "", "Output File Path"=path "", "clConfigOptions"={"TIME_BASE"=1000000, "STN"="Bus_1", "IDCODE"=0, "rdoPolRect"=enum."Rectangular", "rdoFloatInt"=enum."Float", "PHUNIT"=1000000, "rdoFreqDfreq"=enum."Float", "CHNAM"=["VA", "VB", "VC", "V+", "IA", "IB", "IC", "I+"], "chkCfg2Prefix"=TRUE}, "AppPluginINIFilePath"=path "", "AppConfig"=variant, "AppOutput"=variant} ("clBusData"), "BusNumber"=w499) -> (w488:T6)
            n167 = call <vilib>:"Wait at Rendezvous.vi"("error in (no error)"=w495, "ms timeout (-1)"=10000, "rendezvous"=w492) -> ("error out"=w498:errorcluster)  [unwired: 2 in, 2 out]
            n168 = call <userlib>:"AddError.vi"("Severity"="Inform", "Priority"=u8 4, "ErrorArray"=w503, "error in (no error)"=w498) -> ("ErrorArray"=w504:errorcluster[])  [unwired: 6 in, 1 out]
          }
          frame "Stop" {
            w558 = T16 {"Msg"="", "Data"=variant} ("QueueType")
            n169 = property class="BCAdmin.lvclass"(reference=w559) -> ("Accessors:BcQueName"=w554:string)  [unwired: 1 in, 2 out]
            "BcQueName" <- w554
            n170 = call "Enqueue.vi"("Error In"=w545, "Msg"="Exit", "QueRef"=w542) -> ("Error Out"=w544:errorcluster[])  [unwired: 7 in, 1 out]
            n171 = To Variant(anything=w556) -> (Variant=w557:variant)
            n172 = Bundle By Name(cluster=w558, "Data"=w557, "Msg"="Busdata") -> (w551:T16)
            n173 = Obtain Queue(name (unnamed)=w554, element data type=w558, create if not found? (T)=FALSE) -> (queue out=w552:refnum<queue>, error out=w553:errorcluster)  [unwired: 2 in, 1 out]
            n174 = Enqueue Element(queue=w552, element=w551, error in (no error)=w553) -> (error out=w548:errorcluster)  [unwired: 1 in, 2 out]
            n175 = call <userlib>:"AddError.vi"("Severity"="Inform", "Priority"=u8 4, "ErrorArray"=w544, "error in (no error)"=w548) -> ("ErrorArray"=w549:errorcluster[])  [unwired: 6 in, 1 out]
          }
          frame "Exit" {
          }
          frame "Error" {
            n176 = Variant To Data(type=errorcluster[] [], Variant=w567) -> (data=w565:errorcluster[])  [unwired: 1 in, 1 out]
            n177 = for {
              tunnel: w565 -> [w571] mode=indexing
              tunnel: [w570] -> w564
              tunnel: w563 -> [w570]
              w577 = T16 {"Msg"="", "Data"=variant} ("QueueType")
              n178 = To Variant(anything=w571) -> (Variant=w576:variant)
              n179 = Bundle By Name(cluster=w577, "Msg"="Error", "Data"=w576) -> (w574:T16)
              n180 = Obtain Queue(name (unnamed)="BC_Que", element data type=w577, create if not found? (T)=TRUE) -> (queue out=w575:refnum<queue>, error out=w573:errorcluster)  [unwired: 2 in, 1 out]
              n181 = Enqueue Element(queue=w575, element=w574, error in (no error)=w573) -> ()  [unwired: 1 in, 3 out]
            }
            n182 = call <userlib>:"ClearErrors.vi"("ErrorArray"=w564) -> ("ErrorArray"=w568:errorcluster[])  [unwired: 10 in]
          }
          frame Default {
            n183 = property class="BCAdmin.lvclass"(reference=w588) -> ("Accessors:Name"=w587:string)  [unwired: 1 in, 2 out]
            n184 = xnode "Error Ring"("parameter 0"=w582, "parameter 1"=w587) -> ("error out"=w586:errorcluster)
            n185 = call <userlib>:"AddError.vi"("Severity"="Inform", "Priority"=u8 4, "ErrorArray"=w585, "error in (no error)"=w586) -> ("ErrorArray"=w584:errorcluster[])  [unwired: 6 in, 1 out]
          }
        }
      }
    }
    n186 = call "QueueError.vi"("QueRef"=w29, "Error In"=w38) -> ("Error Out"=w37:errorcluster[])  [unwired: 9 in]
    "LastCommand" <- w27
  }
  n187 = property class="BCAdmin.lvclass"(reference=w15) -> (error out=w12:errorcluster, "Accessors:BCRegRef"=w14:refnum<data-value>, "Accessors:BC ID"=w13:i32, "Accessors:First_"=w10:bool)  [unwired: 1 in, 1 out]
  n188 = call "Remove.vi"("error in (no error)"=w12, "BC ID"=w13, "BCReg"=w14) -> ("error out"=w9:errorcluster, "BCReg 2"=w11:refnum<data-value>)  [unwired: 6 in, 1 out]
  n189 = case shown="True" w10 {
    tunnel: w11 -> [_ w601]
    tunnel: w9 -> [w597 w602]
    tunnel: [w597 w598] -> w8
    frame False {
    }
    frame True {
      # "First module waits for the others to be destroyed"
      n190 = while {
        tunnel: w602 -> [w608]
        tunnel: w601 -> [w607]
        tunnel: [w605] -> w600
        tunnel: [w604] -> w599
        stop <- w606 continue-if-true
        # "Wait"
        n191 = call "List.vi"("error in (no error)"=w608, "BCReg"=w607) -> ("error out"=w605:errorcluster, "Found?"=w606:bool, "BCReg"=w604:refnum<data-value>)  [unwired: 4 in, 3 out]
        n192 = Wait (ms)(milliseconds to wait=u32 100) -> ()  [unwired: 1 out]
      }
      n193 = call "Destroy.vi"("error in (no error)"=w600, "BCReg"=w599) -> ("error out"=w598:errorcluster)  [unwired: 9 in]
    }
  }
  n194 = invoke class="VI" method="FP.Close"(error in=w8) -> ()  [unwired: 2 in, 3 out]
